vi "ReceiveString.vi"(8 "error in (no error)":errorcluster, 9 "waiting time ms (-1: forever)":i32, 11 "queue cluster":T1) -> (0 "error out":errorcluster, 1 "new value":bool, 2 "received string":string, 3 "queue cluster out":T1)   [LabVIEW 2014]
uses:
  typedefs/clientStatus.ctl
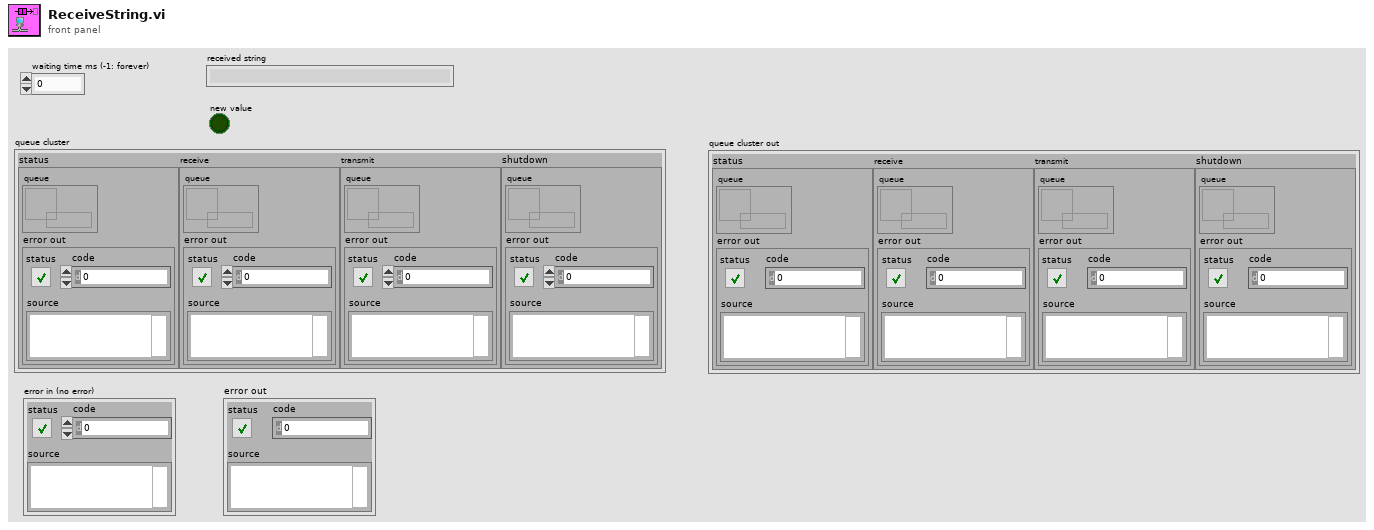
[diagram p1: front panel]
types:
  T1 = cluster{"status":cluster{"queue":refnum<queue>, "error out":errorcluster}, "receive":cluster{"queue":refnum<queue>, "error out":errorcluster}, "transmit":cluster{"queue":refnum<queue>, "error out":errorcluster}, "shutdown":cluster{"queue":refnum<queue>, "error out":errorcluster}}
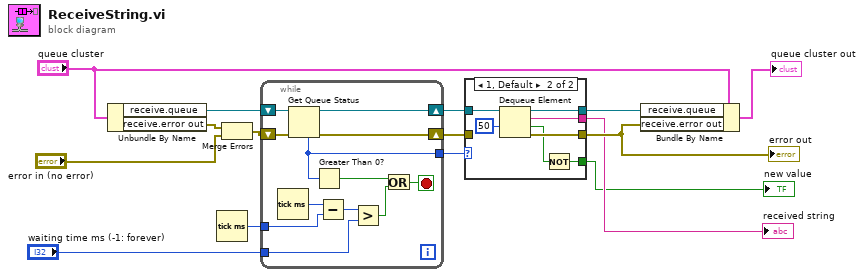
[diagram p0: block diagram]
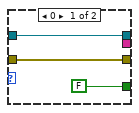
[diagram p2: hidden frame]
diagram:
  n1 = Unbundle By Name("queue cluster") -> ("receive.queue"=w11:refnum<queue>, "receive.error out"=w8:errorcluster)
  n2 = Tick Count (ms)() -> (millisecond timer value=w2:u32)
  n3 = Merge Errors(w8, "error in (no error)") -> (w9:errorcluster)
  n4 = while {
    tunnel: [w22] -> w5
    shift-right: [w26] -> w10
    shift-left: w11 -> [w27]
    shift-right: [w24] -> w6
    shift-left: w9 -> [w25]
    tunnel: w2 -> [w20]
    tunnel: "waiting time ms (-1: forever)" -> [w18]
    stop <- w17 stop-if-true
    n5 = Tick Count (ms)() -> (millisecond timer value=w21:u32)
    n6 = Get Queue Status(queue=w27, error in (no error)=w25) -> (queue out=w26:refnum<queue>, error out=w24:errorcluster, # elements in queue=w22:i32)  [unwired: 1 in, 5 out]
    n7 = Greater Than 0?(x=w22) -> (x > 0?=w23:bool)
    n8 = Subtract(x=w21, y=w20) -> (x-y=w19:u32)
    n9 = Greater?(x=w19, y=w18) -> (0:w16:bool)
    n10 = Or(x=w23, y=w16) -> (x .or. y?=w17:bool)
  }
  n11 = case shown="1, Default" w5 {
    tunnel: [w29 w37] -> w13
    tunnel: [w30 w36] -> w12
    tunnel: [_ w35] -> w4
    tunnel: w10 -> [w30 w34]
    tunnel: w6 -> [w29 _]
    tunnel: [FALSE ("timed out?") w31] -> w3
    frame 0 {
    }
    frame 1, Default {
      n12 = Dequeue Element(queue=w34, timeout in ms (-1)=50) -> (queue out=w36:refnum<queue>, element=w35:string, timed out?=w32:bool, error out=w37:errorcluster)  [unwired: 1 in]
      n13 = Not(x=w32) -> (.not. x?=w31:bool)
    }
  }
  "error out" <- w13
  "received string" <- w4
  "new value" <- w3
  n14 = Bundle By Name(cluster="queue cluster", "receive.queue"=w12, "receive.error out"=w13) -> (→"queue cluster out":T1)
